vi "Build Unregister Status Message.vi"(0 "Target CSM":string, 5 "Source CSM (* as Default)":string="*", 7 "Status":string, 9 "API (* as Default)":string="*") -> (6 "CSM Message String":string)   [LabVIEW 2017, in "Communicable State Machine.lvlib"]
doc: "#### Build Unregister Status Message.vi\n\nConcatenates an unregister status operation message string, with the following format:\n\n //[source-state]@[source-module] >> [response-message]@[response-module] -><unregister>\n status @ Source >> API @ Target -><unregister>\n\nExample: Unbind the download completion message of the downloader module from the start play API of the player module.\n\n // Unbind the download completion message of the downloader module from the start play API of the player module.\n DownloadFinished@Downloader >> StartPlay@Player -><unregister>\n // When executing the message in the player module, Player can be omitted.\n DownloadFinished@Downloader >> StartPlay -><unregister>\n\n> [!NOTE] Message Concatenation API\n> This type of API does not directly send messages, it only concatenates message strings. The strings need to be incorporated into the CSM's state queue and then sent and executed in Parse State Queue++.vi.\n> If you are familiar with CSM rules, you can skip using this type of API and directly type the corresponding message strings and operation strings in the text.\n\n\n<b>Controls</b>\n- <b>Target CSM</b>: The name of the CSM module subscribing to the status.\n- <b>Source CSM (* as Default)</b>: The name of the CSM module issuing the status.\n- <b>Status</b>: The registered status.\n\n<b>Indicators</b>\n- <b>CSM Message String</b>: The concatenated CSM message string."
uses:
  Communicable State Machine.lvlib
  _Shared/CSM Shared.lvlib
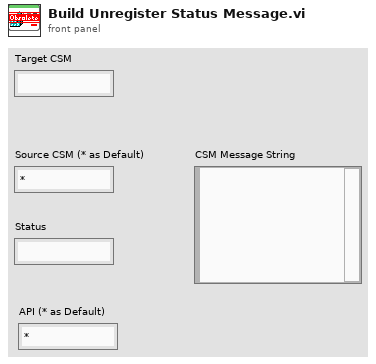
[diagram p1: front panel]
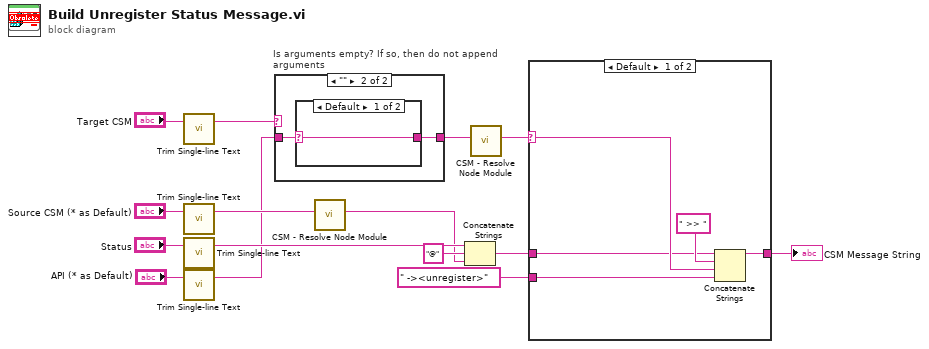
[diagram p0: block diagram]
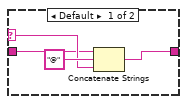
[diagram p2: hidden frame]
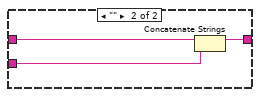
[diagram p4: hidden frame]
diagram:
  n1 = call "Trim Single-line Text.vi"("single-line text"="Target CSM") -> ("trimed text"=w5:string)  [unwired: 2 in]
  n2 = call "Trim Single-line Text.vi"("single-line text"="Source CSM (* as Default)") -> ("trimed text"=w9:string)  [unwired: 2 in]
  n3 = call "Trim Single-line Text.vi"("single-line text"="Status") -> ("trimed text"=w11:string)  [unwired: 2 in]
  n4 = call "Trim Single-line Text.vi"("single-line text"="API (* as Default)") -> ("trimed text"=w3:string)  [unwired: 2 in]
  n5 = case "Is arguments empty? If so, then do not append arguments" shown="\"\"" w5 {
    selector: w5 -> [w17 _]
    tunnel: [w18 w20] -> w4
    tunnel: w3 -> [w16 w21]
    frame Default {
      n6 = Concatenate Strings(w16, "@" ("string"), w17) -> (w18:string)
    }
    frame "" {
      n7 = case shown="Default" w21 {
        selector: w21 -> [w22 _]
        tunnel: [w22 _] -> w20
        frame Default {
        }
        frame "*" {
        }
      }
    }
  }
  n8 = call "CSM - Resolve Node Module.vi"("Node Name"=w9) -> ("CSM Module Name"=w2:string)  [unwired: 10 in]
  n9 = Concatenate Strings(w11, "@" ("string"), w2) -> (w8:string)
  n10 = call "CSM - Resolve Node Module.vi"("Node Name"=w4) -> ("CSM Module Name"=w1:string)  [unwired: 10 in]
  n11 = case shown="Default" w1 {
    selector: w1 -> [w26 _]
    tunnel: [w27 w30] -> w15
    tunnel: w8 -> [w24 w29]
    tunnel: " -><unregister>" ("string") -> [w23 w28]
    frame Default {
      n12 = Concatenate Strings(w24, " >> " ("string"), w26, w23) -> (w27:string)
    }
    frame "" {
      n13 = Concatenate Strings(w29, w28) -> (w30:string)
    }
  }
  "CSM Message String" <- w15
